vi "Initialize.vi"(6 "Synchronize Transferred Files":bool, 8 "error in (no error)":errorcluster, 10 "local path":path) -> (0 "error out":errorcluster, 3 "File Download Controller out":refnum<class "File Download Controller.lvclass">)   [LabVIEW 2020, in "NI_SFTP.lvlib" / "File Download Controller.lvclass"]
uses:
  <vilib>/net/SFTP/API/Support/Download/File/File Download Controller.lvclass
  <vilib>/net/SFTP/API/Support/Download/File/File Download Controller.lvclass/File Download Controller.ctl
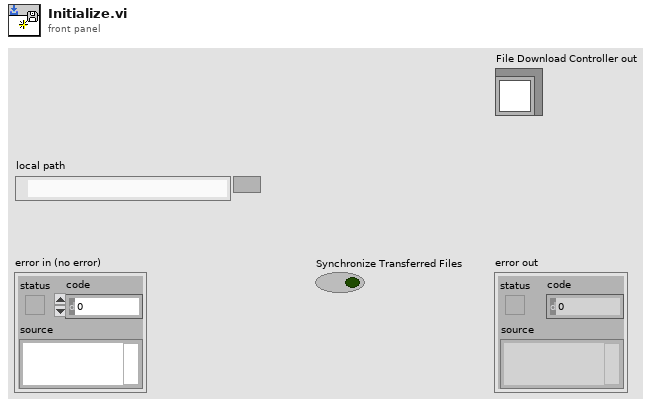
[diagram p1: front panel]
types:
  T1 = enum16{"open", "replace", "create", "open or create", "replace or create", "replace or create with confirmation"}
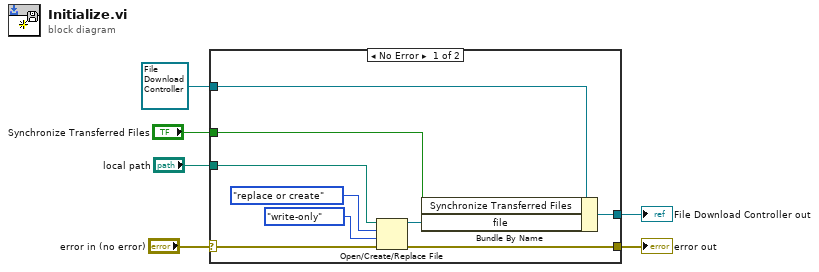
[diagram p0: block diagram]
diagram:
  n1 = case shown="No Error" "error in (no error)" {
    selector: "error in (no error)" -> [w11 w17]
    tunnel: [w10 w17] -> w5
    tunnel: [w9 w16] -> w3
    tunnel: refnum<class "File Download Controller.lvclass"> refnum ("File Download Controller in") -> [w8 w16]
    tunnel: "local path" -> [w13 _]
    tunnel: "Synchronize Transferred Files" -> [w7 _]
    frame No Error {
      n2 = Open/Create/Replace File(file path (use dialog)=w13, error in=w11, operation (0:open)=T1."replace or create", access (0:read/write)=enum16{"read/write", "read-only", "write-only"}."write-only") -> (refnum out=w12:refnum<file>, error out=w10:errorcluster)  [unwired: 2 in, 1 out]
      n3 = Bundle By Name(cluster=w8, "Synchronize Transferred Files"=w7, "file"=w12) -> (w9:refnum<class "File Download Controller.lvclass">)
    }
    frame Error {
    }
  }
  "error out" <- w5
  "File Download Controller out" <- w3
